vi "setAll.vi"(8 "error in (no error)":errorcluster, 9 "Monochromator in":refnum<class "Monochromator.lvclass">, 10 "MonoSetup":T6, 11 "ReadySate in":refnum<class "ReadySate.lvclass">) -> (0 "error out":errorcluster, 1 "Monochromator out":refnum<class "Monochromator.lvclass">, 3 "ReadySate out":refnum<class "ReadySate.lvclass">)   [LabVIEW 2016, in "ReadySate.lvclass"]
uses:
  ReadySate.lvclass
  Monochromator/Monochromator.lvclass
  Typedefs/wavelength.ctl
  Typedefs/slitWidth.ctl
  Typedefs/GratingType.ctl
  Typedefs/slit.ctl
  Typedefs/SlitType.ctl
  Typedefs/SWStatus.ctl
  Typedefs/AckType.ctl
  Commands/CommandFactory/commandList.ctl
  Commands/CommandFactory/CommandFactory.lvclass
panel:
  out "wavelength":T1=400.0
  out "frontExitSlitWidth":T2
  out "fronEntranceSlitWidth":T2
  out "GratingType":T3
  in  "position":T4
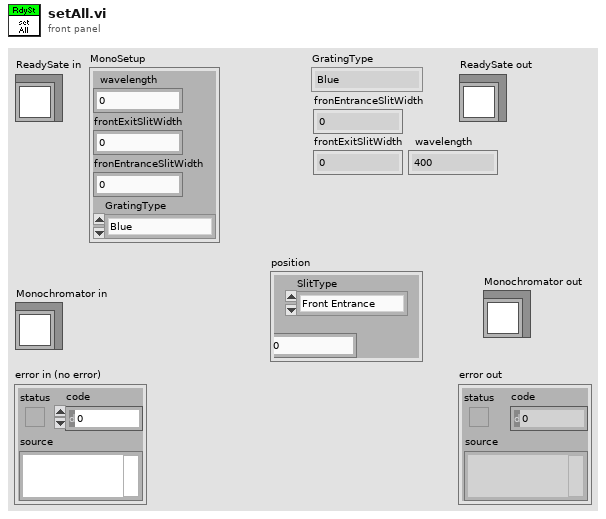
[diagram p1: front panel]
types:
  T1 = typedef "wavelength.ctl" = dbl
  T2 = typedef "slitWidth.ctl" = dbl
  T3 = typedef "GratingType.ctl" = enum16{"Blue", "Red", "Mirror"}
  T4 = typedef "slit.ctl" = cluster{"SlitType":T5, "Width":T2}
  T5 = typedef "SlitType.ctl" = enum16{"Front Entrance", "Side Entrance", "Front Exit", "Side Exit", "First Intermediate", "Second Intermediate"}
  T6 = cluster{"wavelength":T1, "frontExitSlitWidth":T2, "fronEntranceSlitWidth":T2, "GratingType":T3}
  T7 = typedef "commandList.ctl" = enum16{"ChangeSlitWidth", "ChangeWavelendth", "SelectGrating"}
  T8 = typedef "AckType.ctl" = enum16{"OK", "OutOfRange", "Unknown", "Busy", "Rejected"}
  T9 = typedef "SWStatus.ctl" = enum16{"OfflineState", "ReadyState", "SettingUpState", "FaultState"}
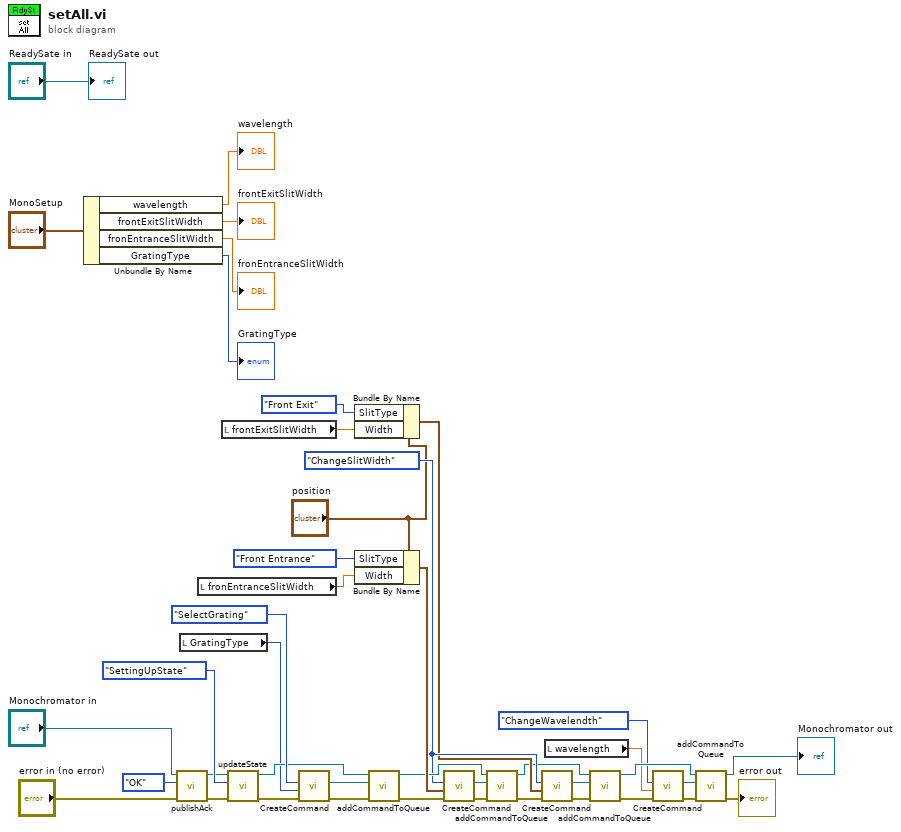
[diagram p0: block diagram]
diagram:
  w20 = commandList."ChangeSlitWidth" ("Command")
  n1 = Unbundle By Name("MonoSetup") -> ("wavelength"=→"wavelength":T1, "frontExitSlitWidth"=→"frontExitSlitWidth":T2, "fronEntranceSlitWidth"=→"fronEntranceSlitWidth":T2, "GratingType"=→"GratingType":T3)
  n2 = call "publishAck.vi"("error in (no error)"="error in (no error)", "Ack"=AckType."OK" ("AckType"), "Monochromator in"="Monochromator in") -> ("error out"=w39:errorcluster, "Monochromator out"=w38:refnum<class "Monochromator.lvclass">)  [unwired: 7 in]
  n3 = local read "GratingType"() -> (w1:T3)
  n4 = local read "fronEntranceSlitWidth"() -> (w2:T2)
  n5 = local read "frontExitSlitWidth"() -> (w3:T2)
  n6 = call "updateState.vi"("error in (no error)"=w39, "SWStatus"=SWStatus."SettingUpState", "Monochromator in"=w38) -> ("error out"=w31:errorcluster, "Monochromator out"=w28:refnum<class "Monochromator.lvclass">)  [unwired: 7 in]
  n7 = call "CreateCommand.vi"("error in (no error)"=w31, "param"=w1, "Command"=commandList."SelectGrating") -> ("error out"=w30:errorcluster, "Command.lvclass"=w29:refnum<class "Command.lvclass">)  [unwired: 6 in, 1 out]
  n8 = Bundle By Name(cluster="position", "SlitType"=SlitType."Front Exit", "Width"=w3) -> (w19:T4)
  n9 = Bundle By Name(cluster="position", "SlitType"=SlitType."Front Entrance", "Width"=w2) -> (w26:T4)
  n10 = call "addCommandToQueue.vi"("error in (no error)"=w30, "Command.lvclass"=w29, "Monochromator in"=w28) -> ("error out"=w25:errorcluster, "Monochromator out"=w24:refnum<class "Monochromator.lvclass">)  [unwired: 7 in]
  n11 = call "CreateCommand.vi"("error in (no error)"=w25, "param"=w26, "Command"=w20) -> ("error out"=w42:errorcluster, "Command.lvclass"=w41:refnum<class "Command.lvclass">)  [unwired: 6 in, 1 out]
  n12 = call "addCommandToQueue.vi"("error in (no error)"=w42, "Command.lvclass"=w41, "Monochromator in"=w24) -> ("error out"=w17:errorcluster, "Monochromator out"=w16:refnum<class "Monochromator.lvclass">)  [unwired: 7 in]
  n13 = call "CreateCommand.vi"("error in (no error)"=w17, "param"=w19, "Command"=w20) -> ("error out"=w21:errorcluster, "Command.lvclass"=w22:refnum<class "Command.lvclass">)  [unwired: 6 in, 1 out]
  n14 = local read "wavelength"() -> (w6:T1)
  n15 = call "addCommandToQueue.vi"("error in (no error)"=w21, "Command.lvclass"=w22, "Monochromator in"=w16) -> ("error out"=w13:errorcluster, "Monochromator out"=w12:refnum<class "Monochromator.lvclass">)  [unwired: 7 in]
  n16 = call "CreateCommand.vi"("error in (no error)"=w13, "param"=w6, "Command"=commandList."ChangeWavelendth") -> ("error out"=w15:errorcluster, "Command.lvclass"=w14:refnum<class "Command.lvclass">)  [unwired: 6 in, 1 out]
  n17 = call "addCommandToQueue.vi"("error in (no error)"=w15, "Command.lvclass"=w14, "Monochromator in"=w12) -> ("error out"=→"error out":errorcluster, "Monochromator out"=→"Monochromator out":refnum<class "Monochromator.lvclass">)  [unwired: 7 in]
  "ReadySate out" <- "ReadySate in"
